vi "MultiSweep_ScanPanel.vi"(8 "error in (no error)":errorcluster caption="entrée d'erreur (pas d'erreur)", 11 "Tools.lvclass":refnum<class "Tools.lvclass">) -> (0 "error out":errorcluster caption="sortie d'erreur", 3 "BaseDevice.lvclass Out":refnum<class "Tools.lvclass">)   [LabVIEW 2019, in "Tools.lvclass"]
uses:
  Tools.lvclass
  C:/Programmes Labview/LabScanV1A/DevicesClass/BaseDevice/BaseDevice.lvclass
panel:
  in  "ModRap":bool caption="Modèle Rapide"
  out "Positions":dbl[](array[numeric])
  in  "Sweeps":u32=1 caption="Sweep Count" min=1 max=100000 step=1
  in  "Stop":bool
  out "Init Program":bool
  # "Multi-Sweep Option"
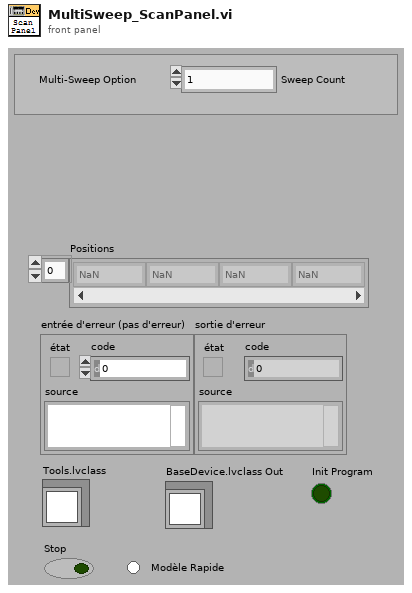
[diagram p1: front panel]
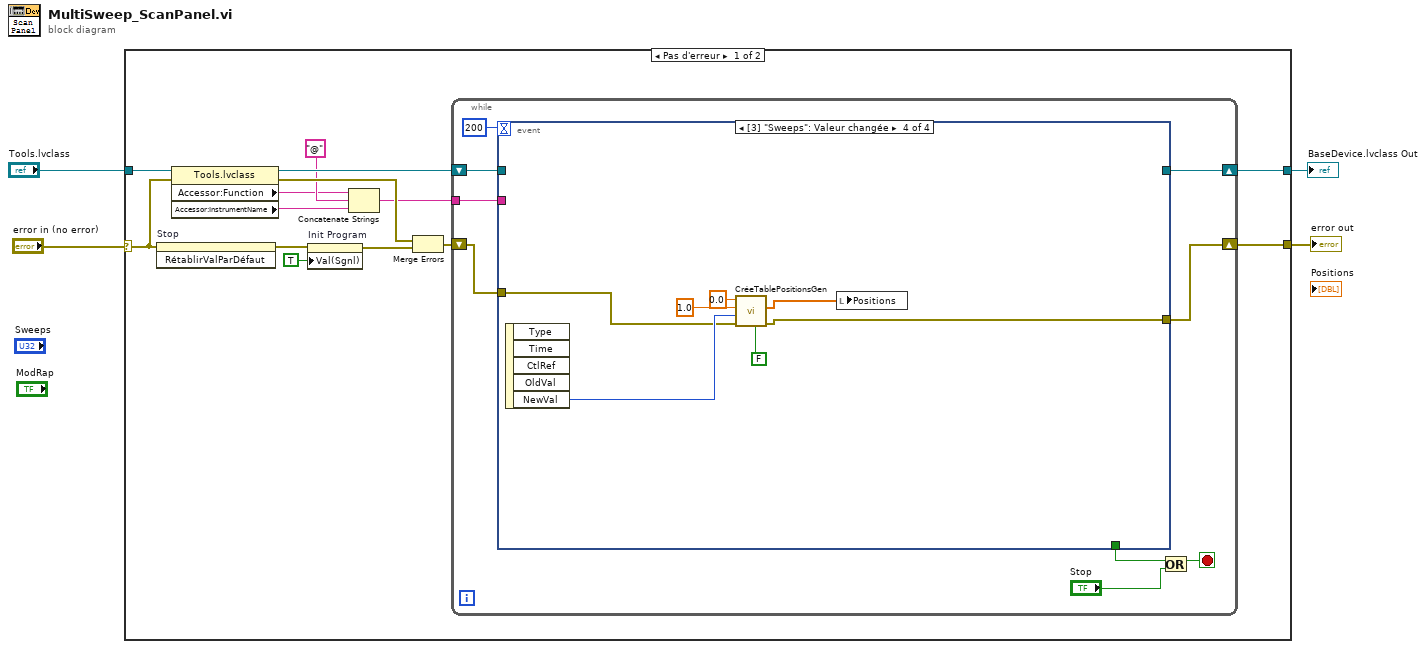
[diagram p0: block diagram]
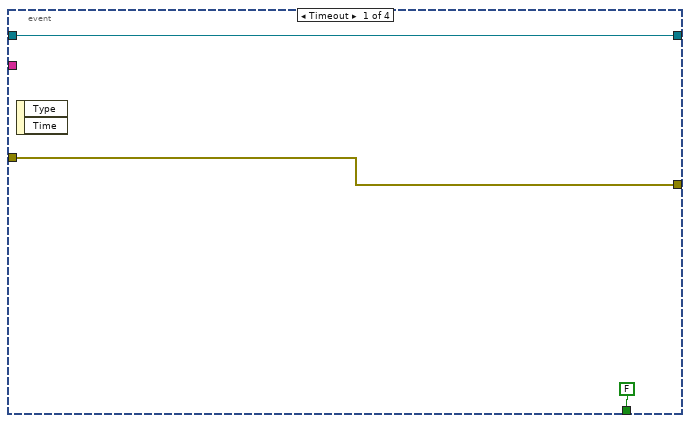
[diagram p2: hidden frame]
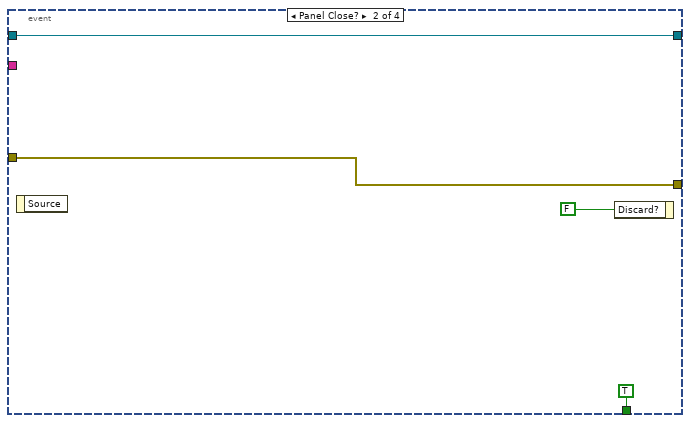
[diagram p3: hidden frame]
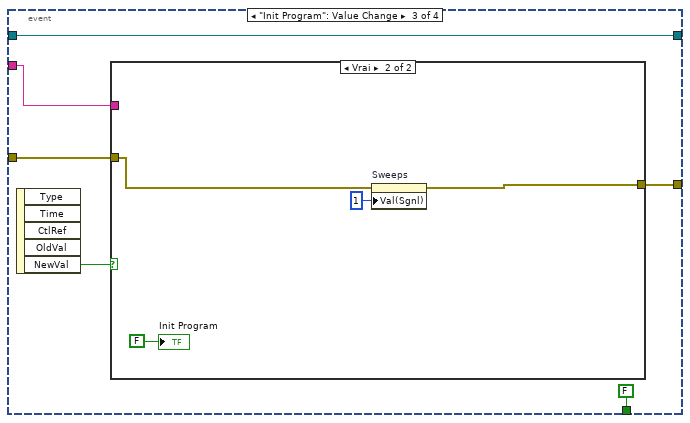
[diagram p4: hidden frame]
diagram:
  n1 = case shown="Pas d'erreur" "error in (no error)" {
    selector: "error in (no error)" -> [w12 w54]
    tunnel: [w18 w54] -> w3
    tunnel: "Tools.lvclass" -> [w17 w53]
    tunnel: [w15 w53] -> w1
    frame No Error {
      n2 = invoke on="Stop" class="Bool (strict)" method="RétablirValParDéfaut"(error in=w12) -> (error out=w14:errorcluster)  [unwired: 2 in, 2 out]
      n3 = property class="Tools.lvclass"(reference=w17, error in=w12) -> (reference out=w13:refnum<class "Tools.lvclass">, error out=w10:errorcluster, "Accessor:Function"=w7:string, "Accessor:InstrumentName"=w6:string)
      n4 = property on="Init Program" class="Bool (strict)"(error in=w14, "Val(Sgnl)"=TRUE ("Valeur (Signalisation)")) -> (error out=w11:errorcluster)  [unwired: 1 in, 1 out]
      n5 = Concatenate Strings(w7, "@" ("chaîne"), w6) -> (w5:string)
      n6 = Merge Errors(w10, w11) -> (w9:errorcluster)
      n7 = while {
        shift-right: [w26] -> w18
        shift-left: w9 -> [w19]
        shift-right: [w23] -> w15
        shift-left: w13 -> [w25]
        tunnel: w5 -> [w20]
        stop <- w22 stop-if-true
        n8 = event shown="[3] \"Sweeps\": Valeur changée" {
          selector: _ -> [_ _ _ _]
          dyn-events: _ -> [_ _ _ _]
          timeout: 200 -> [_ _ _ _]
          tunnel: w19 -> [w28 w32 w39 w48]
          tunnel: [w28 w32 w38 w47] -> w26
          tunnel: w25 -> [w29 w31 w37 _]
          tunnel: [FALSE TRUE FALSE _] -> w24
          tunnel: [w29 w31 w37 _] -> w23
          tunnel: w20 -> [_ _ w35 _]
          event Timeout {
            n9 = event-data() -> ()  [unwired: 1 in, 2 out]
          }
          event Panel Close? {
            n10 = event-data() -> ()  [unwired: 1 in, 1 out]
            n11 = event-data("Discard?"=FALSE ("Rejeter ?")) -> ()  [unwired: 1 in, 1 out]
          }
          event "Init Program": Value Change {
            n12 = event-data() -> ("NewVal"=w40:bool)  [unwired: 1 in, 4 out]
            n13 = case shown="Vrai" w40 {
              tunnel: w35 -> [_ _]
              tunnel: w39 -> [w41 w43]
              tunnel: [w41 w44] -> w38
              frame False {
              }
              frame True {
                n14 = property on="Sweeps" class="NumNb (strict)"(error in=w43, "Val(Sgnl)"=u32 1 ("Value (Signaling)")) -> (error out=w44:errorcluster)  [unwired: 1 in, 1 out]
                "Init Program" <- FALSE
              }
            }
          }
          event "Sweeps": Value Change {
            n15 = event-data() -> ("NewVal"=w50:u32)  [unwired: 1 in, 4 out]
            n16 = call "CréeTablePositionsGen.vi"("IncFin (T)"=FALSE, "error in (no error)"=w48, "Fin"=w50, "Increment"=1.0, "Debut"=0.0) -> ("error out"=w47:errorcluster, "Positions"=w49:dbl[])  [unwired: 4 in, 1 out]
            n17 = local write "Positions"(w49) -> ()
          }
        }
        n18 = Or(x=w24, y="Stop") -> (x .or. y?=w22:bool)
      }
    }
    frame Error {
    }
  }
  "error out" <- w3
  "BaseDevice.lvclass Out" <- w1
